vi "contact sensor.vi"() -> ()   [LabVIEW 2022 SP3]
uses:
  <vilib>/DAQmx/read.llb/DAQmx Read (Analog DBL 1Chan 1Samp).vi
  <vilib>/DAQmx/write.llb/DAQmx Write (Digital Bool 1Line 1Point).vi
  <vilib>/DAQmx/create/channels.llb/DAQmx Create Channel (AI-Voltage-Basic).vi
  <vilib>/DAQmx/create/channels.llb/DAQmx Create Channel (DO-Digital Output).vi
  <vilib>/DAQmx/miscellaneous.llb/DAQmx Fill In Error Info.vi
panel:
  in  "lines":tag
  in  "physical channels":tag
  out "Numeric":i32
  out "Timer":i32
  in  "stop":bool
  out "buzzer":bool
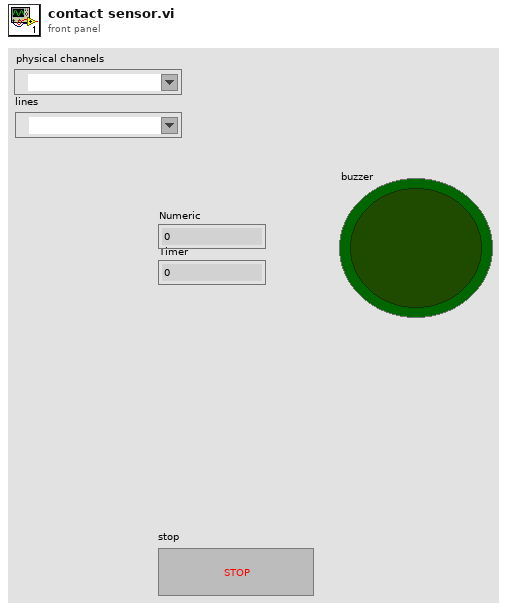
[diagram p1: front panel]
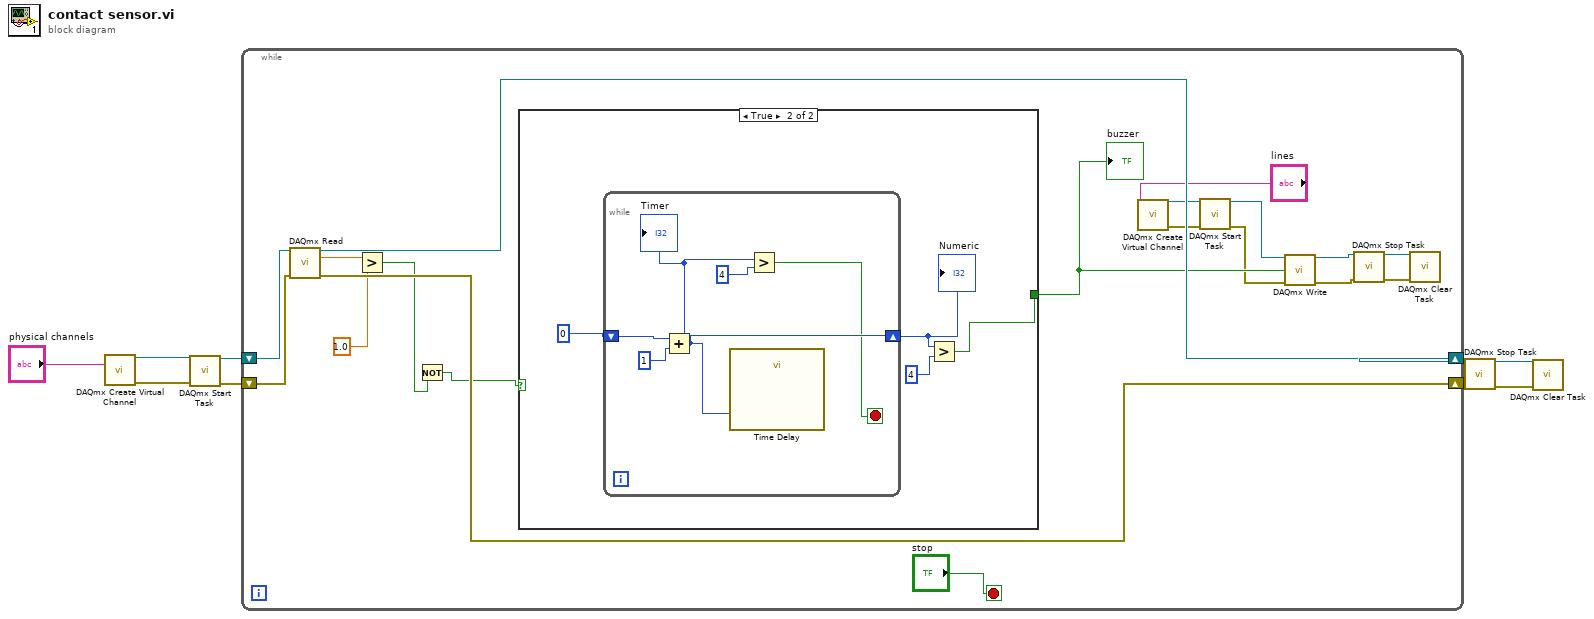
[diagram p0: block diagram]
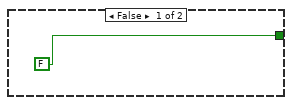
[diagram p2: hidden frame]
diagram:
  n1 = call-poly <vilib>:"DAQmx Create Virtual Channel.vi"("physical channels"="physical channels") -> ("task out"=w9:refnum<k21>, "error out"=w8:errorcluster)  [unwired: 13 in]
  n2 = call <vilib>:"DAQmx Start Task.vi"("task/channels in"=w9, "error in"=w8) -> ("task out"=w7:refnum<k21>, "error out"=w6:errorcluster)  [unwired: 12 in]
  n3 = while {
    shift-right: [w25] -> w3
    shift-left: w7 -> [w27]
    shift-right: [w24] -> w2
    shift-left: w6 -> [w26]
    stop <- "stop" stop-if-true
    n4 = call-poly <vilib>:"DAQmx Read.vi"("task/channels in"=w27, "error in"=w26) -> ("task out"=w25:refnum<k21>, "data"=w23:dbl, "error out"=w24:errorcluster)  [unwired: 11 in]
    n5 = Greater?(x=w23, y=1.0) -> (0:w21:bool)
    n6 = Not(x=w21) -> (.not. x?=w20:bool)
    n7 = case shown="True" w20 {
      tunnel: [FALSE w30] -> w19
      frame False {
      }
      frame True {
        n8 = while {
          shift-right: [w35] -> w33
          shift-left: 0 -> [w38]
          stop <- w34 stop-if-true
          n9 = Add(x=w38, y=1) -> (x+y=w35:i32)
          "Timer" <- w35
          n10 = call "Time Delay"("Delay Time (s)"=w35) -> ()  [unwired: 10 in, 1 out]
          n11 = Greater?(x=w35, y=4) -> (0:w34:bool)
        }
        "Numeric" <- w33
        n12 = Greater?(x=w33, y=4) -> (0:w30:bool)
      }
    }
    "buzzer" <- w19
    n13 = call-poly <vilib>:"DAQmx Create Virtual Channel.vi"("lines"="lines") -> ("task out"=w17:refnum<k21>, "error out"=w16:errorcluster)  [unwired: 13 in]
    n14 = call <vilib>:"DAQmx Start Task.vi"("task/channels in"=w17, "error in"=w16) -> ("task out"=w15:refnum<k21>, "error out"=w14:errorcluster)  [unwired: 12 in]
    n15 = call-poly <vilib>:"DAQmx Write.vi"("task/channels in"=w15, "data"=w19, "error in"=w14) -> ("task out"=w13:refnum<k21>, "error out"=w12:errorcluster)  [unwired: 10 in, 1 out]
    n16 = call <vilib>:"DAQmx Stop Task.vi"("task/channels in"=w13, "error in"=w12) -> ("task out"=w11:refnum<k21>, "error out"=w10:errorcluster)  [unwired: 12 in]
    n17 = call <vilib>:"DAQmx Clear Task.vi"("task in"=w11, "error in"=w10) -> ()  [unwired: 13 in, 1 out]
  }
  n18 = call <vilib>:"DAQmx Stop Task.vi"("task/channels in"=w3, "error in"=w2) -> ("task out"=w5:refnum<k21>, "error out"=w4:errorcluster)  [unwired: 12 in]
  n19 = call <vilib>:"DAQmx Clear Task.vi"("task in"=w5, "error in"=w4) -> ()  [unwired: 13 in, 1 out]
